vi "Stop Core.vi"(10 "final error code":i32, 11 "TDMS-Actor in":refnum<class "TDMS-Actor.lvclass">) -> (3 "TDMS-Actor out":refnum<class "TDMS-Actor.lvclass">)   [LabVIEW 2017, in "BNT_TDMS.lvlib" / "TDMS-Actor.lvclass"]
doc: "(<B>Filename</B>: Actor Framework.lvlib:Actor.lvclass:Stop Core.vi)\n\nDefines what the actor does before it stops. Use the <B>final error code</B> input to determine whether the actor shut down in response to an error.\n\nBy default, this method does nothing. A descendant class may override it to define behavior, such as shutting down any processes the actor initiated in its override of the Actor Core method."
uses:
  TDMS-Actor.lvclass
  CSPP_Core/Actors/CSPP_BaseActor/CSPP_BaseActor.lvclass
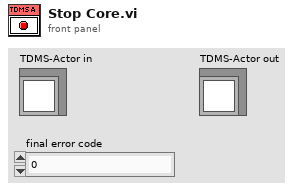
[diagram p1: front panel]
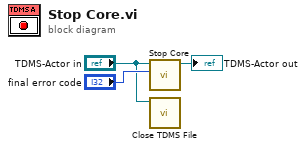
[diagram p0: block diagram]
diagram:
  n1 = call-parent "Stop Core.vi"("final error code"="final error code", "CSPP_BaseActor In"="TDMS-Actor in") -> ("CSPP_BaseActor Out"=→"TDMS-Actor out":refnum<class "TDMS-Actor.lvclass">)  [unwired: 9 in]
  n2 = call "Close TDMS File.vi"("TDMS-Actor in"="TDMS-Actor in") -> ()  [unwired: 9 in, 2 out]
